vi "error.From JSON Tree.vi"(8 "error in (no error)":errorcluster, 10 "JSON Value in":refnum<class "JSON Value.lvclass">, 11 "error in":refnum<class "error.lvclass">) -> (0 "error out":errorcluster, 3 "error out":refnum<class "error.lvclass">)   [LabVIEW 2016, in "error.lvclass"]
uses:
  error.lvclass
  <vilib>/NI/JSON Support for LabVIEW/JSON Value/JSON Value.lvclass
  error.lvclass/error.ctl
  <vilib>/NI/JSON Support for LabVIEW/JSON Value/Object/Get Value/Get Value (Numeric).vi
  <vilib>/NI/JSON Support for LabVIEW/JSON Value/Object/Get Value/Get Value (String).vi
  <vilib>/NI/JSON Support for LabVIEW/JSON Value/Object/Get Value/Get Value (Value).vi
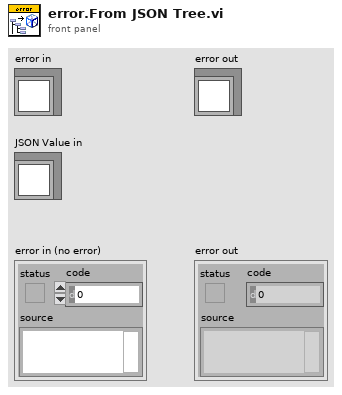
[diagram p1: front panel]
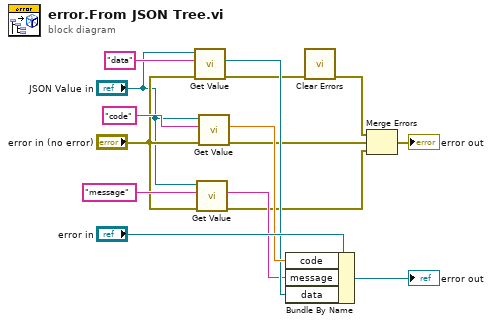
[diagram p0: block diagram]
diagram:
  n1 = call-poly <vilib>:"Get Value.vi"("error in (no error)"="error in (no error)", "key"="data" ("Parameter Name"), "JSON Value in"="JSON Value in") -> ("error out"=w3:errorcluster, "JSON Value out"=w10:refnum<class "JSON Value.lvclass">)  [unwired: 7 in]
  n2 = call-poly <vilib>:"Get Value.vi"("error in (no error)"="error in (no error)", "key"="message" ("Parameter Name"), "JSON Value in"="JSON Value in") -> ("error out"=w5:errorcluster, "value"=w8:string)  [unwired: 7 in]
  n3 = call-poly <vilib>:"Get Value.vi"("error in (no error)"="error in (no error)", "key"="code" ("Parameter Name"), "JSON Value in"="JSON Value in") -> ("error out"=w7:errorcluster, "value"=w12:dbl)  [unwired: 7 in]
  n4 = Bundle By Name(cluster="error in", "code"=w12, "message"=w8, "data"=w10) -> (→"error out":refnum<class "error.lvclass">)
  n5 = call <vilib>:"Clear Errors.vi"("error in (no error)"=w3) -> ("error out"=w2:errorcluster)  [unwired: 5 in, 1 out]
  n6 = Merge Errors(w2, w7, w5) -> (→"error out":errorcluster)
